vi "Enqueue Data.vi"(8 "error in":errorcluster, 11 "Data":string[][](array[string])) -> (0 "error out":errorcluster, 3 "overflow?":bool)   [LabVIEW 2025, in "Automotive Ethernet Bus Monitor UI.lvlib"]
doc: "Write data into the Table Buffer."
uses:
  Automotive Ethernet Bus Monitor UI.lvlib
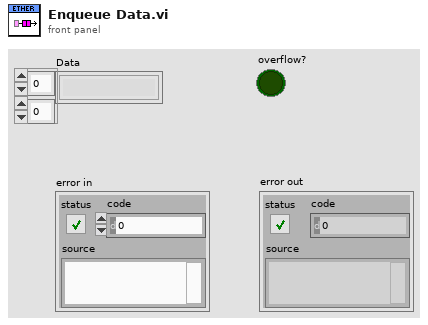
[diagram p1: front panel]
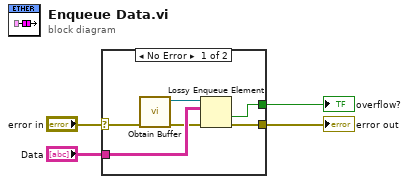
[diagram p0: block diagram]
diagram:
  n1 = case shown="No Error" "error in" {
    selector: "error in" -> [w6 w11]
    tunnel: [w10 w11] -> w2
    tunnel: "Data" -> [w9 _]
    tunnel: [w8 _] -> w1
    frame No Error {
      n2 = call "Obtain Buffer.vi"("error in (no error)"=w6) -> ("error out"=w7:errorcluster, "Table Queue"=w5:refnum<queue>)  [unwired: 9 in]
      n3 = Lossy Enqueue Element(queue=w5, element=w9, error in (no error)=w7) -> (overflow?=w8:bool, error out=w10:errorcluster)  [unwired: 2 out]
    }
    frame Error {
    }
  }
  "error out" <- w2
  "overflow?" <- w1
